vi "Combo Box,Ring, Enum, String.vi"() -> ()   [LabVIEW 2022 SP3]
panel:
  in  "Combo Box":string(combo)
  in  "Text Ring":u16(ring) items=["Ansi C", "C++", "ýthon", "C#"]
  in  "Menu Ring":u16(ring) items=["Piña", "Limon", "Durazno", "Manzana"]
  in  "Paises":enum16{"Peru", "Mexico", "Colombia", "Ecuador"}(ring)
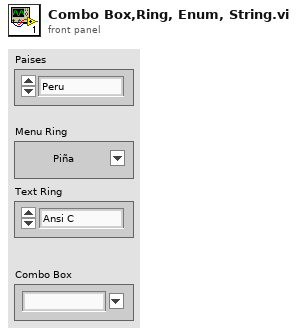
[diagram p1: front panel]
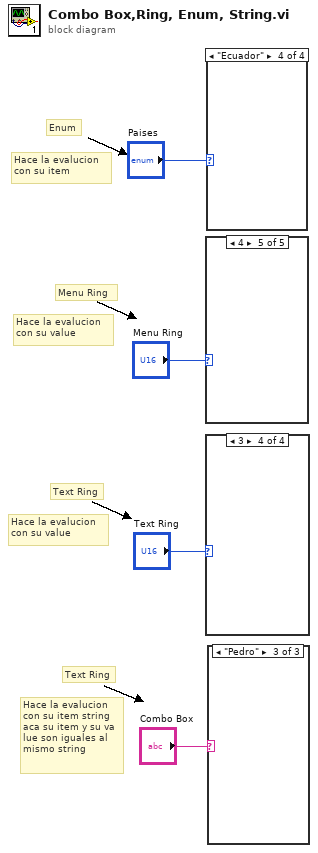
[diagram p0: block diagram]
diagram:
  # "Hace la evalucion \ncon su item string\naca su item y su va\nlue son iguales al\nmismo string"
  # "Text Ring"
  # "Hace la evalucion \ncon su value"
  # "Text Ring"
  # "Hace la evalucion \ncon su value"
  # "Hace la evalucion \ncon su item"
  # "Menu Ring"
  # "Enum"
  n1 = case shown="4" "Menu Ring" {
    frame 0, Default {
    }
    frame 1 {
    }
    frame 2 {
    }
    frame 3 {
    }
    frame 4 {
    }
  }
  n2 = case shown="3" "Text Ring" {
    frame 0, Default {
    }
    frame 1 {
    }
    frame 2 {
    }
    frame 3 {
    }
  }
  n3 = case shown="\"Ecuador\"" "Paises" {
    frame "Peru", Default {
    }
    frame "Mexico" {
    }
    frame "Colombia" {
    }
    frame "Ecuador" {
    }
  }
  n4 = case shown="\"Pedro\"" "Combo Box" {
    frame "Carlos", Default {
    }
    frame "Javier" {
    }
    frame "Pedro" {
    }
  }
